vi "lv_opencv_demo.vi"() -> ()   [LabVIEW 2021]
uses:
  cmake-build-debug/detect_lay.dll
panel:
  out "1/n捻距":dbl(graph)
  out "直径":dbl(graph)
  out "像素直方图":dbl
  out "摆幅":dbl
  out "耗时(s)":dbl
  out "直径(像素)":dbl
  out "角度(度)":dbl
  out "1/n捻距(像素)":dbl
  in  "img_Path":path
  out "roi":T1(plugin-control)
  out "Original":T1(plugin-control)
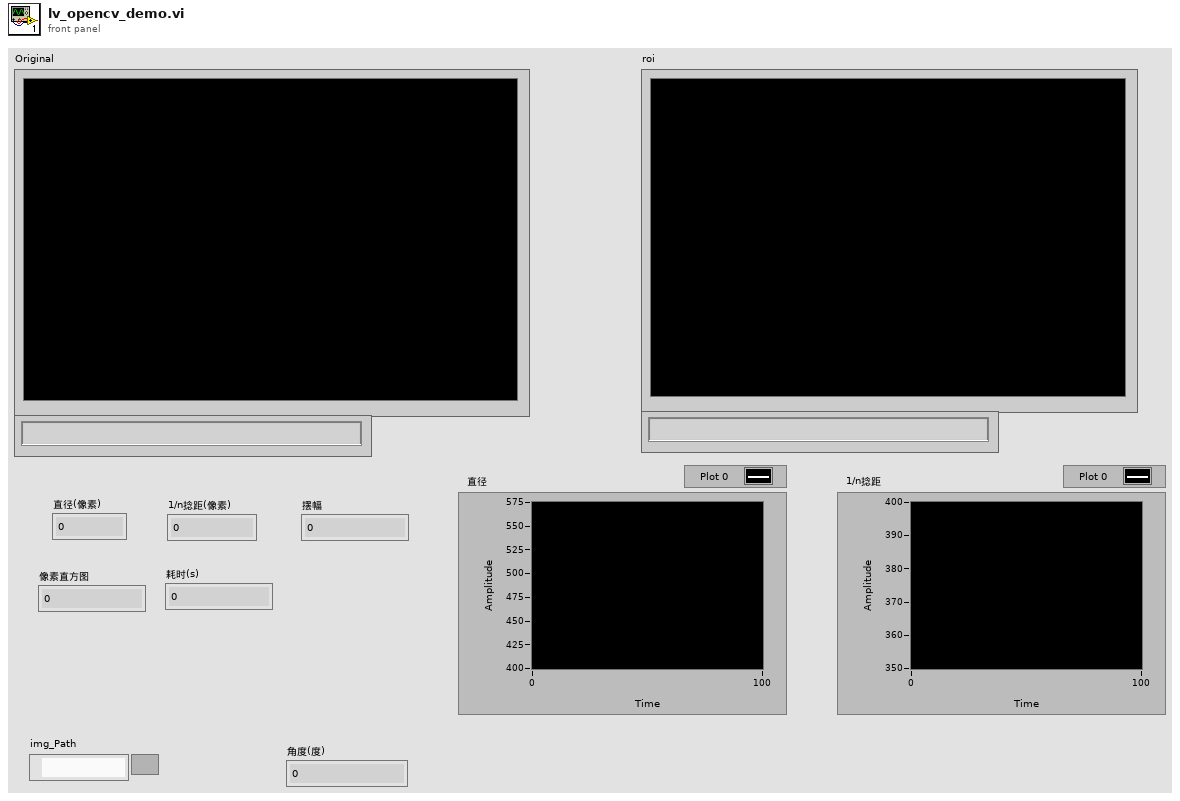
[diagram p1: front panel]
types:
  T1 = typedef "IMAQ Image.ctl" = refnum<image>
  T2 = typedef "Image Type" = u32
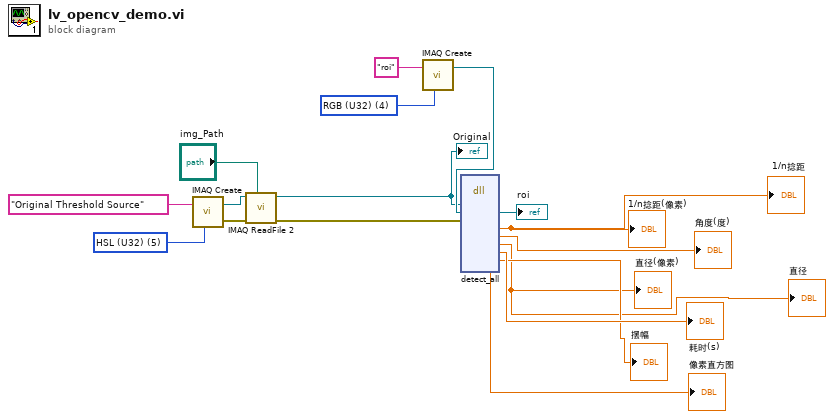
[diagram p0: block diagram]
diagram:
  w6 = T2 4 items=["Grayscale (U8)", "Grayscale (I16)", "Grayscale (SGL)", "Complex (CSG)", "RGB (U32)", "HSL (U32)", "RGB (U64)", "Grayscale (U16)"] ("Image Type")
  w14 = T2 5 items=["Grayscale (U8)", "Grayscale (I16)", "Grayscale (SGL)", "Complex (CSG)", "RGB (U32)", "HSL (U32)", "RGB (U64)", "Grayscale (U16)"] ("Image Type")
  n1 = call "IMAQ Create"("Image Name"="Original Threshold Source", "Image Type"=w14) -> ("New Image"=w16:T1, "error out"=w15:errorcluster)  [unwired: 3 in]
  n2 = call "IMAQ ReadFile 2"("File Path"="img_Path", "error in (no error)"=w15, "Image"=w16) -> ("error out"=w3:errorcluster, "Image Out"=w4:T1)  [unwired: 4 in, 3 out]
  "Original" <- w4
  n3 = call "IMAQ Create"("Image Name"="roi", "Image Type"=w6) -> ("New Image"=w5:T1)  [unwired: 3 in, 1 out]
  n4 = dll-call lib="D:/projects/cppProjects/detect_lay/cmake-build-debug/detect_lay.dll" fn="detect_all"("sourceHandle_src"=w4, "destHandle"=w5, "errorHandle"=w3) -> ("destHandle"=→"roi":T1, "lay"=→"1/n捻距(像素)" →"1/n捻距":dbl, "angle"=→"角度(度)":sgl, "diameter"=→"直径(像素)" →"直径":dbl, "time"=→"耗时(s)":dbl, "swing"=→"摆幅":dbl, "arr"=→"像素直方图":sgl)  [unwired: 12 in, 2 out]
